vi "Serial_communication_simple.vi"() -> ()   [LabVIEW 2015]
uses:
  MFC_Address.ctl
  Program Files (x86)/National Instruments/LabVIEW 2015/examples/Instrument IO/Serial/support/Serial - Settings.ctl
  <vilib>/Instr/_visa.llb/VISA Configure Serial Port (Instr).vi
panel:
  out "숫자형 인디케이터":dbl
  in  "Command":string
  out "flow":sgl
  out "Error Out":errorcluster caption="에러 출력"
  in  "Error In":errorcluster caption="에러 입력"
  in  "VISA resource name":refnum<visa-resource-name>="COM1"
  in  "delay before read (ms)":u32=500
  out "bytes read":u32
  in  "Serial Settings":T1={"baud rate"=9600, "data bits"=8, "parity"=enum."None", "stop bits"=10, "flow control"=0} {"flow control" items=["None"=0, "XON/XOFF"=1, "RTS/CTS"=2, "DTR/DSR"=4]; "stop bits" items=["1.0"=10, "1.5"=15, "2.0"=20]; "data bits" min=5 max=8 step=1; "baud rate" items=["75"=75, "110"=110, "134"=134, "150"=150, "300"=300, "600"=600, "1200"=1200, "1800"=1800, "2400"=2400, "4800"=4800, "7200"=7200, "9600"=9600, "14400"=14400, "19200"=19200, "28800"=28800, "38400"=38400, "56000"=56000, "57600"=57600, "115200"=115200, "128000"=128000, "230400"=230400]}
  out "Response":T2
  out "반환 카운트":u32
  in  "Enable Termination\nChar (T)":bool=TRUE caption="종료 문자\n활성화(참)"
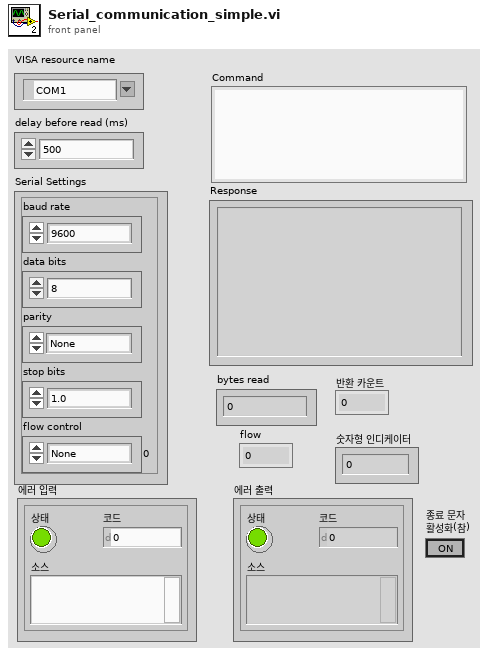
[diagram p1: front panel]
types:
  T1 = typedef "Serial - Settings.ctl" = cluster{"baud rate":u32, "data bits":u16, "parity":enum16{"None", "Odd", "Even", "Mark", "Space"}, "stop bits":u16, "flow control":u16}
  T2 = typedef "MFC_Address.ctl" = string
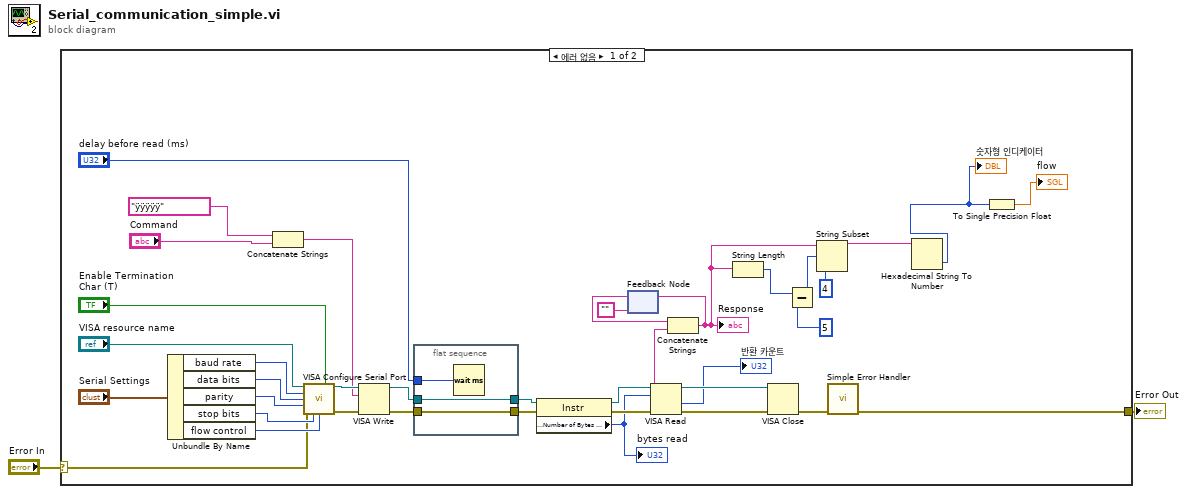
[diagram p0: block diagram]
diagram:
  n1 = case shown="에러 없음" "Error In" {
    selector: "Error In" -> [w16 w44]
    tunnel: [w15 w44] -> w1
    frame No Error {
      n2 = Unbundle By Name("Serial Settings") -> ("baud rate"=w25:u32, "data bits"=w24:u16, "parity"=w23:enum16{"None", "Odd", "Even", "Mark", "Space"}, "stop bits"=w22:u16, "flow control"=w21:u16)
      n3 = Concatenate Strings("ÿÿÿÿÿ" ("문자열"), "Command") -> (w6:string)
      n4 = call-poly "VISA Configure Serial Port"("VISA resource name"="VISA resource name", "Enable Termination\nChar (T)"="Enable Termination\nChar (T)", "baud rate (9600)"=w25, "data bits (8)"=w24, "parity (0:none)"=w23, "error in (no error)"=w16, "stop bits (10: 1 bit)"=w22, "flow control (0:none)"=w21) -> ("VISA resource name out"=w38:refnum<visa-resource-name>, "error out"=w39:errorcluster)  [unwired: 1 in, 5 out]
      n5 = VISA Write(VISA resource name=w38, write buffer=w6, error in (no error)=w39) -> (VISA resource name out=w32:refnum<visa-resource-name>, error out=w34:errorcluster)  [unwired: 1 out]
      n6 = flat-sequence {
        tunnel: w34 -> [w42]
        tunnel: [w42] -> w33
        tunnel: w32 -> [w41]
        tunnel: [w41] -> w31
        tunnel: "delay before read (ms)" -> [w43]
        frame #0 {
          n7 = Wait (ms)(milliseconds to wait=w43) -> ()  [unwired: 1 out]
        }
      }
      n8 = property class="Instr"(reference=w31, error in=w33) -> (reference out=w29:refnum<visa-resource-name>, error out=w28:errorcluster, "Serial Settings:Number of Bytes at Serial Port"=w27:u32)
      "bytes read" <- w27
      n9 = feedback #1("") -> (w20:string)
      n10 = VISA Read(VISA resource name=w29, byte count=w27, error in (no error)=w28) -> (VISA resource name out=w36:refnum<visa-resource-name>, read buffer=w18:string, return count=→"반환 카운트":u32, error out=w37:errorcluster)
      n11 = Concatenate Strings(w20, w18) -> (w13:string)
      "Response" <- w13
      n12 = feedback-in #1(w13) -> ()
      n13 = String Length(string=w13) -> (length=w12:i32)
      n14 = VISA Close(VISA resource name=w36, error in (no error)=w37) -> (error out=w35:errorcluster)
      n15 = Subtract(x=w12, y=5) -> (x-y=w10:i32)
      n16 = String Subset(string=w13, offset (0)=w10, length (rest)=4 ("길이(나머지)")) -> (substring=w8:string)
      n17 = call <vilib>:"Simple Error Handler.vi"("error in (no error)"=w35) -> ("error out"=w15:errorcluster)  [unwired: 1 in, 7 out]
      n18 = Hexadecimal String To Number(string=w8) -> (number=w3:u32)  [unwired: 2 in, 1 out]
      "숫자형 인디케이터" <- w3
      n19 = To Single Precision Float(number=w3) -> (single precision float=→"flow":sgl)
    }
    frame Error {
    }
  }
  "Error Out" <- w1
